vi "Release-cameras.vi"(8 "error in":errorcluster, 11 "Data ref. in":refnum<data-value>) -> (0 "error IO":errorcluster, 3 "Data ref.":refnum<data-value>)   [LabVIEW 2013, in "CameraVision.lvlib" / "CV-Main.lvclass"]
uses:
  CV-Main.lvclass
  CV-Main.lvclass/CV-Main.ctl
  Configuration/CV-Configuration.lvclass/CV-Configuration.ctl
  UI/Module-states.ctl
  Hardware/Camera/Camera.lvclass
  Read Config params.vi
  Configuration/Read Camera array.vi
  Configuration/Read Camera status.vi
  Configuration/CV-Configuration.lvclass
  UI/CV-UI.lvclass
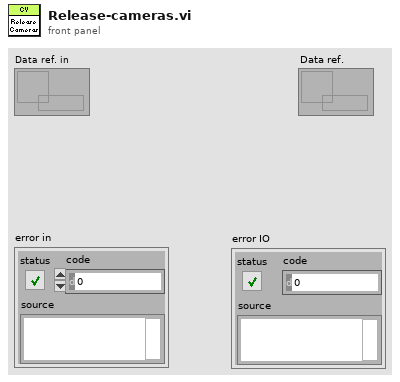
[diagram p1: front panel]
types:
  T1 = typedef "CameraVision.lvlib/CV-UI.lvclass/Module-states.ctl" = enum16{"Inactive", "Active", "Data-loss", "Error", "Simulation", "Synchronizing", "Initialized", "Released"}
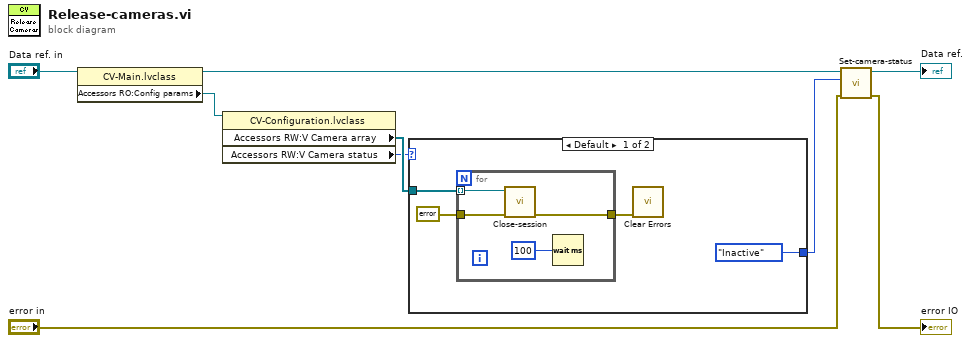
[diagram p0: block diagram]
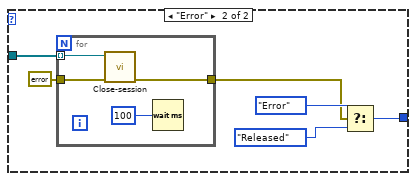
[diagram p2: hidden frame]
diagram:
  n1 = property class="CV-Main.lvclass"(reference="Data ref. in") -> (reference out=w8:refnum<data-value>, "Accessors RO:Config params"=w5:refnum<data-value>)  [unwired: 1 in, 1 out]
  n2 = property class="CV-Configuration.lvclass"(reference=w5) -> ("Accessors RW:V Camera array"=w7:refnum<class "Camera.lvclass">[], "Accessors RW:V Camera status"=w6:T1)  [unwired: 1 in, 2 out]
  n3 = case shown="Default" w6 {
    tunnel: w7 -> [w12 w23]
    tunnel: [Module-states."Inactive" ("Grabber status") w20] -> w1
    frame Default {
      n4 = for {
        tunnel: w12 -> [w16] mode=indexing
        tunnel: errorcluster {"status"=FALSE, "code"=0, "source"=""} ("error out") -> [w15]
        tunnel: [w14] -> w11
        n5 = call-dynamic "Close-session.vi"("error in (no error)"=w15, "Camera in"=w16) -> ("error out"=w14:errorcluster)  [unwired: 6 in, 3 out]
        n6 = Wait (ms)(milliseconds to wait=u32 100 ("millisecond multiple")) -> ()  [unwired: 1 out]
      }
      n7 = call <vilib>:"Clear Errors.vi"("error in (no error)"=w11) -> ()  [unwired: 6 in, 1 out]
    }
    frame "Error" {
      n8 = for {
        tunnel: w23 -> [w26] mode=indexing
        tunnel: errorcluster {"status"=FALSE, "code"=0, "source"=""} ("error out") -> [w25]
        tunnel: [w24] -> w19
        n9 = call-dynamic "Close-session.vi"("error in (no error)"=w25, "Camera in"=w26) -> ("error out"=w24:errorcluster)  [unwired: 6 in, 3 out]
        n10 = Wait (ms)(milliseconds to wait=u32 100 ("millisecond multiple")) -> ()  [unwired: 1 out]
      }
      n11 = Select(t=Module-states."Error" ("Grabber status"), s=w19, f=Module-states."Released" ("Grabber status")) -> (s? t:f=w20:T1)
    }
  }
  n12 = call "Set-camera-status.vi"("error in"="error in", "Cam. status in"=w1, "Data ref. in"=w8) -> ("error IO"=→"error IO":errorcluster, "Data ref."=→"Data ref.":refnum<data-value>)  [unwired: 6 in, 1 out]
